vi "Raster_Scan_FSRS.vi"() -> ()   [LabVIEW 2014] (continued)
{"X"=544.0, "Y"=0.9978545183540273}, {"X"=545.0, "Y"=0.9978954802718253}, {"X"=546.0, "Y"=0.9978847126029841}, {"X"=547.0, "Y"=0.9986282274099947}, {"X"=548.0, "Y"=0.9985592746779094}, {"X"=549.0, "Y"=0.9984101644173519}, {"X"=550.0, "Y"=0.9981985424776665}, {"X"=551.0, "Y"=0.998426104497088}, {"X"=552.0, "Y"=0.9985691286987668}, {"X"=553.0, "Y"=0.9979689171383916}, {"X"=554.0, "Y"=0.9982460987713048}, {"X"=555.0, "Y"=0.998121473974186}, {"X"=556.0, "Y"=0.9977379675030132}, {"X"=557.0, "Y"=0.998243375619955}, {"X"=558.0, "Y"=0.998132359067814}, {"X"=559.0, "Y"=0.9983256230790136}, {"X"=560.0, "Y"=0.9980172261705131}, {"X"=561.0, "Y"=0.9984771190185349}, {"X"=562.0, "Y"=0.9979225481535584}, {"X"=563.0, "Y"=0.9981209325830508}, {"X"=564.0, "Y"=0.9981205014531911}, {"X"=565.0, "Y"=0.9985116348563284}, {"X"=566.0, "Y"=0.9985313300015474}, {"X"=567.0, "Y"=0.9985618507511264}, {"X"=568.0, "Y"=0.9980731056228417}, {"X"=569.0, "Y"=0.99777584834941}, {"X"=570.0, "Y"=0.9983204895779979}, {"X"=571.0, "Y"=0.9979093460943547}, {"X"=572.0, "Y"=0.9974202665539573}, {"X"=573.0, "Y"=0.9974138091852186}, {"X"=574.0, "Y"=0.99811669466617}, {"X"=575.0, "Y"=0.9981038738953151}, {"X"=576.0, "Y"=0.9977082372079878}, {"X"=577.0, "Y"=0.9980030461884963}, {"X"=578.0, "Y"=0.9980034114768427}, {"X"=579.0, "Y"=0.9982364510217848}, {"X"=580.0, "Y"=0.9979325576022529}, {"X"=581.0, "Y"=0.9977734094940269}, {"X"=582.0, "Y"=0.9981140314943433}, {"X"=583.0, "Y"=0.9979539107254143}, {"X"=584.0, "Y"=0.997655931871743}, {"X"=585.0, "Y"=0.9972543054374033}, {"X"=586.0, "Y"=0.9969317121833642}, {"X"=587.0, "Y"=0.9968443093625065}, {"X"=588.0, "Y"=0.9966413383535035}, {"X"=589.0, "Y"=0.9960249116592703}, {"X"=590.0, "Y"=0.9963089300738579}, {"X"=591.0, "Y"=0.9961840817664352}, {"X"=592.0, "Y"=0.9963553748195709}, {"X"=593.0, "Y"=0.9962705798119079}, {"X"=594.0, "Y"=0.99670571106408}, {"X"=595.0, "Y"=0.9964327341637447}, {"X"=596.0, "Y"=0.9965823060297267}, {"X"=597.0, "Y"=0.9968535449226337}, {"X"=598.0, "Y"=0.9965539588406062}, {"X"=599.0, "Y"=0.9961449417496469}, {"X"=600.0, "Y"=0.9965984047900572}, {"X"=601.0, "Y"=0.9962586900884038}, {"X"=602.0, "Y"=0.9962103374424071}, {"X"=603.0, "Y"=0.9954906975090069}, {"X"=604.0, "Y"=0.9957365549620107}, {"X"=605.0, "Y"=0.9963388156166715}, {"X"=606.0, "Y"=0.9965861993129}, {"X"=607.0, "Y"=0.9974232683784019}, {"X"=608.0, "Y"=0.9992020432658635}, {"X"=609.0, "Y"=1.00039405639493}, {"X"=610.0, "Y"=1.0013783401587335}, {"X"=611.0, "Y"=1.0033275791215845}, {"X"=612.0, "Y"=1.0047939581934993}, {"X"=613.0, "Y"=1.0072483446876968}, {"X"=614.0, "Y"=1.008871757151934}, {"X"=615.0, "Y"=1.0110282901417909}, {"X"=616.0, "Y"=1.013371337166815}, {"X"=617.0, "Y"=1.0151009747430668}, {"X"=618.0, "Y"=1.0176425122069255}, {"X"=619.0, "Y"=1.0197495431887913}, {"X"=620.0, "Y"=1.0224688407170561}, {"X"=621.0, "Y"=1.0247490900420204}, {"X"=622.0, "Y"=1.0276990459376787}, {"X"=623.0, "Y"=1.0296095041094517}, {"X"=624.0, "Y"=1.0333078315506532}, {"X"=625.0, "Y"=1.0362685626177792}, {"X"=626.0, "Y"=1.038924641533091}, {"X"=627.0, "Y"=1.041572265389145}, {"X"=628.0, "Y"=1.0435587138867348}, {"X"=629.0, "Y"=1.0464705907166}, {"X"=630.0, "Y"=1.0490032103492144}, {"X"=631.0, "Y"=1.050504978522211}, {"X"=632.0, "Y"=1.0528251069017325}, {"X"=633.0, "Y"=1.0534239144824968}, {"X"=634.0, "Y"=1.0549006626365562}, {"X"=635.0, "Y"=1.0550592680988555}, {"X"=636.0, "Y"=1.0549458189191194}, {"X"=637.0, "Y"=1.0549779342343906}, {"X"=638.0, "Y"=1.0539315349680067}, {"X"=639.0, "Y"=1.0542361563716711}, {"X"=640.0, "Y"=1.0534478719509481}, {"X"=641.0, "Y"=1.052399132550848}, {"X"=642.0, "Y"=1.0514082647686147}, {"X"=643.0, "Y"=1.0504137881143336}, {"X"=644.0, "Y"=1.0488047450457352}, {"X"=645.0, "Y"=1.0477270368509513}, {"X"=646.0, "Y"=1.045690156385211}, {"X"=647.0, "Y"=1.0432872265980713}, {"X"=648.0, "Y"=1.0410317960687832}, {"X"=649.0, "Y"=1.0379447532276453}, {"X"=650.0, "Y"=1.0348336539420064}, {"X"=651.0, "Y"=1.0315576847668324}, {"X"=652.0, "Y"=1.028862670120101}, {"X"=653.0, "Y"=1.0258567044055389}, {"X"=654.0, "Y"=1.0230131849598842}, {"X"=655.0, "Y"=1.0209637506857185}, {"X"=656.0, "Y"=1.0181556258277114}, {"X"=657.0, "Y"=1.0160814779436314}, {"X"=658.0, "Y"=1.0136796020817032}, {"X"=659.0, "Y"=1.0120789147322529}, {"X"=660.0, "Y"=1.0104539182883303}, {"X"=661.0, "Y"=1.008677968134813}, {"X"=662.0, "Y"=1.0068674140821063}, {"X"=663.0, "Y"=1.005416554572116}, {"X"=664.0, "Y"=1.004418287860281}, {"X"=665.0, "Y"=1.0026019255081793}, {"X"=666.0, "Y"=1.001755051681397}, {"X"=667.0, "Y"=1.0007427244836384}, {"X"=668.0, "Y"=1.000212255121392}, {"X"=669.0, "Y"=1.0001516680923108}, {"X"=670.0, "Y"=1.0002951868519772}, {"X"=671.0, "Y"=0.9997153062030121}, {"X"=672.0, "Y"=0.9996816416219783}, {"X"=673.0, "Y"=0.9998761682577347}, {"X"=674.0, "Y"=0.9992615693650128}, {"X"=675.0, "Y"=1.000324398030068}, {"X"=676.0, "Y"=0.9999570200209895}, {"X"=677.0, "Y"=1.0000117210295363}, {"X"=678.0, "Y"=1.0000634134316824}, {"X"=679.0, "Y"=1.0001331522973944}, {"X"=680.0, "Y"=1.0004081949275365}, {"X"=681.0, "Y"=0.9998829901655063}, {"X"=682.0, "Y"=1.000187544558325}, {"X"=683.0, "Y"=1.0003801314997531}, {"X"=684.0, "Y"=1.0003149177046684}, {"X"=685.0, "Y"=0.9998517079056821}, {"X"=686.0, "Y"=1.0004100893131052}, {"X"=687.0, "Y"=1.0000016158957639}, {"X"=688.0, "Y"=1.0006017898810222}, {"X"=689.0, "Y"=1.0005718409574569}, {"X"=690.0, "Y"=1.0007007698411632}, {"X"=691.0, "Y"=1.000506938601441}, {"X"=692.0, "Y"=1.0000772828380353}, {"X"=693.0, "Y"=1.0005686668319205}, {"X"=694.0, "Y"=1.0009164301763613}, {"X"=695.0, "Y"=1.0004825673685438}, {"X"=696.0, "Y"=1.000543465394958}, {"X"=697.0, "Y"=1.00084754089509}, {"X"=698.0, "Y"=1.0006573921442272}, {"X"=699.0, "Y"=1.0008281174083582}, {"X"=700.0, "Y"=1.001000500464312}, {"X"=701.0, "Y"=1.0005876920760894}, {"X"=702.0, "Y"=1.000993095286034}, {"X"=703.0, "Y"=1.00056708158604}, {"X"=704.0, "Y"=1.0006259107721924}, {"X"=705.0, "Y"=1.0007697612854025}, {"X"=706.0, "Y"=1.000978106387117}, {"X"=707.0, "Y"=1.0007664078085046}, {"X"=708.0, "Y"=1.0011454626210547}, {"X"=709.0, "Y"=1.0011091615448482}, {"X"=710.0, "Y"=1.001056081943534}, {"X"=711.0, "Y"=1.0012334014028355}, {"X"=712.0, "Y"=1.0011837250778726}, {"X"=713.0, "Y"=1.000916622339644}, {"X"=714.0, "Y"=1.0012569862720535}, {"X"=715.0, "Y"=1.0009918254170156}, {"X"=716.0, "Y"=1.0007201726153137}, {"X"=717.0, "Y"=1.0011288843771156}, {"X"=718.0, "Y"=1.0008681092115939}, {"X"=719.0, "Y"=1.0009798044664915}, {"X"=720.0, "Y"=1.001112027329558}, {"X"=721.0, "Y"=1.0010204159387182}, {"X"=722.0, "Y"=1.0006192087669428}, {"X"=723.0, "Y"=1.0012939973290147}, {"X"=724.0, "Y"=1.0007005394153075}, {"X"=725.0, "Y"=1.0009357538518868}, {"X"=726.0, "Y"=1.0014740988896245}, {"X"=727.0, "Y"=1.0010121967650842}, {"X"=728.0, "Y"=1.0016954160298988}, {"X"=729.0, "Y"=1.0011144874969538}, {"X"=730.0, "Y"=1.000975865976058}, {"X"=731.0, "Y"=1.0011789828226225}, {"X"=732.0, "Y"=1.0011893085482935}, {"X"=733.0, "Y"=1.0011614230048504}, {"X"=734.0, "Y"=1.0011976845828305}, {"X"=735.0, "Y"=1.0011581305715418}, {"X"=736.0, "Y"=1.0010556075044197}, {"X"=737.0, "Y"=1.000937577300871}, {"X"=738.0, "Y"=1.0009325997585012}, {"X"=739.0, "Y"=1.0007734996223567}, {"X"=740.0, "Y"=1.0008682847275774}, {"X"=741.0, "Y"=1.0009267272013356}, {"X"=742.0, "Y"=1.0009202446313439}, {"X"=743.0, "Y"=1.0011286199467828}, {"X"=744.0, "Y"=1.0009420307972523}, {"X"=745.0, "Y"=1.0011039647090711}, {"X"=746.0, "Y"=1.0009233724169802}, {"X"=747.0, "Y"=1.0007503724260123}, {"X"=748.0, "Y"=1.0008308485115536}, {"X"=749.0, "Y"=1.0009287533631965}, {"X"=750.0, "Y"=1.0007719252489964}, {"X"=751.0, "Y"=1.0008692070915899}, {"X"=752.0, "Y"=1.0008582123092458}, {"X"=753.0, "Y"=1.0005798712787062}, {"X"=754.0, "Y"=1.0009749912624057}, {"X"=755.0, "Y"=1.0009132421180837}, {"X"=756.0, "Y"=1.0006067695791088}, {"X"=757.0, "Y"=1.0006890331168343}, {"X"=758.0, "Y"=1.0008962054677861}, {"X"=759.0, "Y"=1.0005844554606693}, {"X"=760.0, "Y"=1.0008238897141335}, {"X"=761.0, "Y"=1.0008713716200581}, {"X"=762.0, "Y"=1.000462698368419}, {"X"=763.0, "Y"=1.00038551560003}, {"X"=764.0, "Y"=1.0005740364073854}, {"X"=765.0, "Y"=1.0010253429662304}, {"X"=766.0, "Y"=1.0003632657418395}, {"X"=767.0, "Y"=1.000567308693705}, {"X"=768.0, "Y"=1.000286790348577}, {"X"=769.0, "Y"=1.0004665761914815}, {"X"=770.0, "Y"=1.000168483840905}, {"X"=771.0, "Y"=1.000152637463018}, {"X"=772.0, "Y"=1.000214242192368}, {"X"=773.0, "Y"=1.0003869867588742}, {"X"=774.0, "Y"=1.0005376955714191}, {"X"=775.0, "Y"=1.0004800558745468}, {"X"=776.0, "Y"=1.0005707911790136}, {"X"=777.0, "Y"=0.9997487173368662}, {"X"=778.0, "Y"=1.0004505353589024}, {"X"=779.0, "Y"=1.0006358048732418}, {"X"=780.0, "Y"=1.0006913500666466}, {"X"=781.0, "Y"=1.0000594857246996}, {"X"=782.0, "Y"=1.000202033665066}, {"X"=783.0, "Y"=1.0005896258602271}, {"X"=784.0, "Y"=0.9998116953891122}, {"X"=785.0, "Y"=1.0000030368836728}, {"X"=786.0, "Y"=0.9999692468282858}, {"X"=787.0, "Y"=0.9996749236190133}, {"X"=788.0, "Y"=0.9999528813725637}, {"X"=789.0, "Y"=0.9996934968232128}, {"X"=790.0, "Y"=1.0001246386179192}, {"X"=791.0, "Y"=1.000121231707337}, {"X"=792.0, "Y"=1.0003574387962126}, {"X"=793.0, "Y"=0.9998897647562817}, {"X"=794.0, "Y"=0.999991814875864}, {"X"=795.0, "Y"=0.9999717796372998}, {"X"=796.0, "Y"=0.9999164248339153}, {"X"=797.0, "Y"=1.0000472803501612}, {"X"=798.0, "Y"=1.0003096307675872}, {"X"=799.0, "Y"=0.9995521439215307}, {"X"=800.0, "Y"=0.9998268441921865}, {"X"=801.0, "Y"=0.9997823002205563}, {"X"=802.0, "Y"=0.9997914401002861}, {"X"=803.0, "Y"=0.999436665219622}, {"X"=804.0, "Y"=0.9996389638963711}, {"X"=805.0, "Y"=0.999683035386018}, {"X"=806.0, "Y"=0.9999043749665063}, {"X"=807.0, "Y"=0.999872375868445}, {"X"=808.0, "Y"=0.9995564412851898}, {"X"=809.0, "Y"=0.9997146784363528}, {"X"=810.0, "Y"=0.9992468990944221}, {"X"=811.0, "Y"=0.9999100681507468}, {"X"=812.0, "Y"=0.9996803844051546}, {"X"=813.0, "Y"=0.999812736922049}, {"X"=814.0, "Y"=0.9999079641000937}, {"X"=815.0, "Y"=0.9995712757348625}, {"X"=816.0, "Y"=0.9999753952150852}, {"X"=817.0, "Y"=0.9996161230527898}, {"X"=818.0, "Y"=0.9999692827506793}, {"X"=819.0, "Y"=0.9997854374958309}, {"X"=820.0, "Y"=0.9997379623488489}, {"X"=821.0, "Y"=0.9997951408693897}, {"X"=822.0, "Y"=0.9996005558855302}, {"X"=823.0, "Y"=0.9996013042279536}, {"X"=824.0, "Y"=0.9994527699487141}, {"X"=825.0, "Y"=0.9994611971332913}, {"X"=826.0, "Y"=0.9995943046267404}, {"X"=827.0, "Y"=0.9993996315141247}, {"X"=828.0, "Y"=0.999466764473007}, {"X"=829.0, "Y"=0.9997275186993784}, {"X"=830.0, "Y"=0.9994655220422562}, {"X"=831.0, "Y"=0.9999217304306618}, {"X"=832.0, "Y"=0.9995485361962716}, {"X"=833.0, "Y"=0.9998723066127978}, {"X"=834.0, "Y"=0.9995042794915885}, {"X"=835.0, "Y"=0.9995245056820103}, {"X"=836.0, "Y"=0.9991550561955388}, {"X"=837.0, "Y"=0.9996330482905573}, {"X"=838.0, "Y"=0.9999634602317182}, {"X"=839.0, "Y"=0.999554498145934}, {"X"=840.0, "Y"=0.9993969166206773}, {"X"=841.0, "Y"=0.9994570922088231}, {"X"=842.0, "Y"=0.9994160747857141}, {"X"=843.0, "Y"=0.9995563480657043}, {"X"=844.0, "Y"=0.9999575192332566}, {"X"=845.0, "Y"=0.9994287267946973}, {"X"=846.0, "Y"=0.9997828708624986}, {"X"=847.0, "Y"=0.9997294658304303}, {"X"=848.0, "Y"=0.9997987491676308}, {"X"=849.0, "Y"=0.9998366805189256}, {"X"=850.0, "Y"=0.9998421980321909}, {"X"=851.0, "Y"=0.9997708290381001}, {"X"=852.0, "Y"=0.9997571893188337}, {"X"=853.0, "Y"=0.9999425601459052}, {"X"=854.0, "Y"=0.999591626867619}, {"X"=855.0, "Y"=0.9997575945123861}, {"X"=856.0, "Y"=0.9998259214523023}, {"X"=857.0, "Y"=0.9998524142922023}, {"X"=858.0, "Y"=0.9998214349671982}, {"X"=859.0, "Y"=0.9996982431382163}, {"X"=860.0, "Y"=1.000006724215444}, {"X"=861.0, "Y"=0.9997226946982664}, {"X"=862.0, "Y"=1.0001222798385383}, {"X"=863.0, "Y"=0.9997723680899672}, {"X"=864.0, "Y"=1.0004691521323734}, {"X"=865.0, "Y"=0.9995317329722564}, {"X"=866.0, "Y"=0.9999706638370606}, {"X"=867.0, "Y"=0.9999485081385426}, {"X"=868.0, "Y"=1.0002513015681866}, {"X"=869.0, "Y"=1.0001094834288995}, {"X"=870.0, "Y"=1.0000796165289747}, {"X"=871.0, "Y"=1.0001052236277999}, {"X"=872.0, "Y"=1.0004937362292834}, {"X"=873.0, "Y"=1.000013590642817}, {"X"=874.0, "Y"=1.0003573287643348}, {"X"=875.0, "Y"=1.0004525481711148}, {"X"=876.0, "Y"=0.9999755900094128}, {"X"=877.0, "Y"=1.0003964124631561}, {"X"=878.0, "Y"=1.0005363708541122}, {"X"=879.0, "Y"=1.0004557806466459}, {"X"=880.0, "Y"=1.000733510349076}, {"X"=881.0, "Y"=1.0002652087127946}, {"X"=882.0, "Y"=1.0003971179645745}, {"X"=883.0, "Y"=1.0006048161778602}, {"X"=884.0, "Y"=1.0005937878882152}, {"X"=885.0, "Y"=1.000476561139529}, {"X"=886.0, "Y"=1.0004827953448545}, {"X"=887.0, "Y"=1.000421392196533}, {"X"=888.0, "Y"=1.0003776494746428}, {"X"=889.0, "Y"=1.0002335494105024}, {"X"=890.0, "Y"=1.0005818770177213}, {"X"=891.0, "Y"=1.000556169743754}, {"X"=892.0, "Y"=1.0005142471348096}, {"X"=893.0, "Y"=1.0006009804720526}, {"X"=894.0, "Y"=1.000462567319067}, {"X"=895.0, "Y"=1.0004232511191642}, {"X"=896.0, "Y"=1.0002985391510821}, {"X"=897.0, "Y"=1.000563080763287}, {"X"=898.0, "Y"=1.0003985868488332}, {"X"=899.0, "Y"=1.0005921693519613}, {"X"=900.0, "Y"=1.0005517113896354}, {"X"=901.0, "Y"=1.0004511874507864}, {"X"=902.0, "Y"=1.0003164509105338}, {"X"=903.0, "Y"=1.0006514699992903}, {"X"=904.0, "Y"=1.0004630517353699}, {"X"=905.0, "Y"=1.0003696899849848}, {"X"=906.0, "Y"=1.0000750343598261}, {"X"=907.0, "Y"=1.0001652803283667}, {"X"=908.0, "Y"=1.0005821961595347}, {"X"=909.0, "Y"=1.0000753056610996}, {"X"=910.0, "Y"=1.0008381429666606}, {"X"=911.0, "Y"=1.0002009630275162}, {"X"=912.0, "Y"=1.0000090046202812}, {"X"=913.0, "Y"=1.000357217161673}, {"X"=914.0, "Y"=1.0005551947210591}, {"X"=915.0, "Y"=1.0006019344688362}, {"X"=916.0, "Y"=1.0003157102839864}, {"X"=917.0, "Y"=1.0006539638821532}, {"X"=918.0, "Y"=1.0004523550286122}, {"X"=919.0, "Y"=1.0004362081948674}, {"X"=920.0, "Y"=1.0004658381122902}, {"X"=921.0, "Y"=1.0005032431132526}, {"X"=922.0, "Y"=1.0006496135004674}, {"X"=923.0, "Y"=1.000421409515476}, {"X"=924.0, "Y"=1.00029741571484}, {"X"=925.0, "Y"=1.0003752604308016}, {"X"=926.0, "Y"=1.0000674401177483}, {"X"=927.0, "Y"=1.000752504898771}, {"X"=928.0, "Y"=1.0004265589119117}, {"X"=929.0, "Y"=1.000277485793791}, {"X"=930.0, "Y"=1.000143732812286}, {"X"=931.0, "Y"=1.000586072623539}, {"X"=932.0, "Y"=1.0003218460655414}, {"X"=933.0, "Y"=1.000253779745408}, {"X"=934.0, "Y"=0.9999684895073191}, {"X"=935.0, "Y"=1.0000553542910315}, {"X"=936.0, "Y"=1.0004387435193063}, {"X"=937.0, "Y"=1.0005796043709154}, {"X"=938.0, "Y"=1.0002239035981928}, {"X"=939.0, "Y"=1.0005100497007755}, {"X"=940.0, "Y"=1.000276926115426}, {"X"=941.0, "Y"=1.0005393916224292}, {"X"=942.0, "Y"=1.0003102290640964}, {"X"=943.0, "Y"=1.0004510828201474}, {"X"=944.0, "Y"=1.0004024270555596}, {"X"=945.0, "Y"=1.0003071722234138}, {"X"=946.0, "Y"=1.0003479438286045}, {"X"=947.0, "Y"=1.0006054265939661}, {"X"=948.0, "Y"=1.0004341205130898}, {"X"=949.0, "Y"=1.0005543120812839}, {"X"=950.0, "Y"=1.0004009168011205}, {"X"=951.0, "Y"=1.0006692411711766}, {"X"=952.0, "Y"=1.0005684966442148}, {"X"=953.0, "Y"=1.0002059600051625}, {"X"=954.0, "Y"=1.0004913192089357}, {"X"=955.0, "Y"=1.0003185704962576}, {"X"=956.0, "Y"=1.0003571139773684}, {"X"=957.0, "Y"=1.0004792329148344}, {"X"=958.0, "Y"=1.0007107646312456}, {"X"=959.0, "Y"=1.0003472703541094}, {"X"=960.0, "Y"=1.00055060436529}, {"X"=961.0, "Y"=1.0002969671654476}, {"X"=962.0, "Y"=1.0002867873822994}, {"X"=963.0, "Y"=1.0003786420047431}, {"X"=964.0, "Y"=1.0003682377805028}, {"X"=965.0, "Y"=1.0005896761650959}, {"X"=966.0, "Y"=1.0003457782727248}, {"X"=967.0, "Y"=1.0006909634949526}, {"X"=968.0, "Y"=1.0001113405044946}, {"X"=969.0, "Y"=1.0003299278640605}, {"X"=970.0, "Y"=1.0006022370584085}, {"X"=971.0, "Y"=1.0002903312662772}, {"X"=972.0, "Y"=1.0005061770542671}, {"X"=973.0, "Y"=1.0004220088897762}, {"X"=974.0, "Y"=1.00062971722216}, {"X"=975.0, "Y"=1.0003765492341081}, {"X"=976.0, "Y"=1.0004592871043285}, {"X"=977.0, "Y"=1.000514847516494}, {"X"=978.0, "Y"=1.0003467113971076}, {"X"=979.0, "Y"=1.0002069450901978}, {"X"=980.0, "Y"=1.0005040498159148}, {"X"=981.0, "Y"=1.000138336954979}, {"X"=982.0, "Y"=1.000390235537673}, {"X"=983.0, "Y"=1.000504818092738}, {"X"=984.0, "Y"=1.0002436968618853}, {"X"=985.0, "Y"=1.0004223209898575}, {"X"=986.0, "Y"=1.0002155513016582}, {"X"=987.0, "Y"=1.0001190993872675}, {"X"=988.0, "Y"=1.000394310225494}, {"X"=989.0, "Y"=1.0004553646966243}, {"X"=990.0, "Y"=1.0001042595318252}, {"X"=991.0, "Y"=1.000235823625573}, {"X"=992.0, "Y"=1.0002616383711564}, {"X"=993.0, "Y"=1.0003022919280078}, {"X"=994.0, "Y"=1.000557447133573}, {"X"=995.0, "Y"=1.0002431232712843}, {"X"=996.0, "Y"=1.000407779249664}, {"X"=997.0, "Y"=1.0001910030091277}, {"X"=998.0, "Y"=1.0000811448918354}, {"X"=999.0, "Y"=1.000409690537901}, {"X"=1000.0, "Y"=1.0003398218940822}, {"X"=1001.0, "Y"=1.000204245610935}, {"X"=1002.0, "Y"=1.00018533413993}, {"X"=1003.0, "Y"=1.000302314225904}, {"X"=1004.0, "Y"=1.0002923742421739}, {"X"=1005.0, "Y"=1.000309364574194}, {"X"=1006.0, "Y"=1.0000426923874066}, {"X"=1007.0, "Y"=1.0004618206725626}, {"X"=1008.0, "Y"=1.0003141108219815}, {"X"=1009.0, "Y"=1.0005023576969727}, {"X"=1010.0, "Y"=1.0003544772082134}, {"X"=1011.0, "Y"=1.0004524090568325}, {"X"=1012.0, "Y"=1.0001465182625013}, {"X"=1013.0, "Y"=1.0002729209887085}, {"X"=1014.0, "Y"=1.0003807048184004}, {"X"=1015.0, "Y"=1.0000934145436753}, {"X"=1016.0, "Y"=1.000523744822201}, {"X"=1017.0, "Y"=1.0003810050685418}, {"X"=1018.0, "Y"=1.0001897441615633}, {"X"=1019.0, "Y"=1.0000433790093919}, {"X"=1020.0, "Y"=1.0002344668735443}, {"X"=1021.0, "Y"=1.0000743430369654}, {"X"=1022.0, "Y"=1.0005123321725913}, {"X"=1023.0, "Y"=0.9999867984833275}, {"X"=1024.0, "Y"=1.00028886416398}, {"X"=1025.0, "Y"=0.9999976564025252}, {"X"=1026.0, "Y"=1.000147489191159}, {"X"=1027.0, "Y"=1.0001021283303542}, {"X"=1028.0, "Y"=1.0004207742794315}, {"X"=1029.0, "Y"=1.0003511315237172}, {"X"=1030.0, "Y"=1.0002740488978419}, {"X"=1031.0, "Y"=1.0005715604928058}, {"X"=1032.0, "Y"=1.0000849731377497}, {"X"=1033.0, "Y"=1.000664325326948}, {"X"=1034.0, "Y"=1.0002715158858457}, {"X"=1035.0, "Y"=1.0004068426842052}, {"X"=1036.0, "Y"=1.0003341226908409}, {"X"=1037.0, "Y"=1.0003845014598438}, {"X"=1038.0, "Y"=1.000382059982626}, {"X"=1039.0, "Y"=1.0002566925098917}, {"X"=1040.0, "Y"=1.0004394237268197}, {"X"=1041.0, "Y"=1.0003796791309603}, {"X"=1042.0, "Y"=1.0005573908410998}, {"X"=1043.0, "Y"=1.0003274420534478}, {"X"=1044.0, "Y"=1.000649864733999}, {"X"=1045.0, "Y"=1.0001894757842382}, {"X"=1046.0, "Y"=1.0003630377518922}, {"X"=1047.0, "Y"=1.0007311125223617}, {"X"=1048.0, "Y"=1.0003937967302898}, {"X"=1049.0, "Y"=1.0004660000627263}, {"X"=1050.0, "Y"=1.000370743171769}, {"X"=1051.0, "Y"=1.0003895018697897}, {"X"=1052.0, "Y"=1.0003660457840664}, {"X"=1053.0, "Y"=1.0006618337709967}, {"X"=1054.0, "Y"=1.0004746367542625}, {"X"=1055.0, "Y"=1.0006470220462966}, {"X"=1056.0, "Y"=1.000336358127014}, {"X"=1057.0, "Y"=1.0004776161543254}, {"X"=1058.0, "Y"=1.0005350625396425}, {"X"=1059.0, "Y"=1.0007114086431932}, {"X"=1060.0, "Y"=1.0005461150814388}, {"X"=1061.0, "Y"=1.0001568330212558}, {"X"=1062.0, "Y"=1.0006049675270903}, {"X"=1063.0, "Y"=1.0008072532845746}, {"X"=1064.0, "Y"=1.0007899340972959}, {"X"=1065.0, "Y"=1.0003705264800233}, {"X"=1066.0, "Y"=1.000663501831443}, {"X"=1067.0, "Y"=1.0003968148498383}, {"X"=1068.0, "Y"=1.0004410295865593}, {"X"=1069.0, "Y"=1.000990825072581}, {"X"=1070.0, "Y"=1.0007069226291818}, {"X"=1071.0, "Y"=1.0009074944245333}, {"X"=1072.0, "Y"=1.000986596814561}, {"X"=1073.0, "Y"=1.0006469461319005}, {"X"=1074.0, "Y"=1.0006961161864978}, {"X"=1075.0, "Y"=1.0009206991231543}, {"X"=1076.0, "Y"=1.0004970130469557}, {"X"=1077.0, "Y"=1.0008897415638358}, {"X"=1078.0, "Y"=1.0004689157169488}, {"X"=1079.0, "Y"=1.0008271789537952}, {"X"=1080.0, "Y"=1.0005958642457493}, {"X"=1081.0, "Y"=1.0006627201543532}, {"X"=1082.0, "Y"=1.000911669123488}, {"X"=1083.0, "Y"=1.0007669752129835}, {"X"=1084.0, "Y"=1.0007869594284737}, {"X"=1085.0, "Y"=1.0008017239957097}, {"X"=1086.0, "Y"=1.0006641645030927}, {"X"=1087.0, "Y"=1.0004027285217332}, {"X"=1088.0, "Y"=1.0005489411934159}, {"X"=1089.0, "Y"=1.0007225000918056}, {"X"=1090.0, "Y"=1.0009034474609535}, {"X"=1091.0, "Y"=1.000700412495902}, {"X"=1092.0, "Y"=1.000559530919639}, {"X"=1093.0, "Y"=1.000504483593376}, {"X"=1094.0, "Y"=1.0006442407338632}, {"X"=1095.0, "Y"=1.0007664841012642}, {"X"=1096.0, "Y"=1.000595386528809}, {"X"=1097.0, "Y"=1.0006037218552855}, {"X"=1098.0, "Y"=1.0006076992023385}, {"X"=1099.0, "Y"=1.0008559458938961}, {"X"=1100.0, "Y"=1.0003974508855653}, {"X"=1101.0, "Y"=1.000520661832493}, {"X"=1102.0, "Y"=1.0007578111149742}, {"X"=1103.0, "Y"=1.0008950719357999}, {"X"=1104.0, "Y"=1.0005845587993554}, {"X"=1105.0, "Y"=1.0004975573787183}, {"X"=1106.0, "Y"=1.0005630280187985}, {"X"=1107.0, "Y"=1.0004865609128089}, {"X"=1108.0, "Y"=1.0005512637747156}, {"X"=1109.0, "Y"=1.0002904477140733}, {"X"=1110.0, "Y"=1.0007674753310123}, {"X"=1111.0, "Y"=1.00048425912666}, {"X"=1112.0, "Y"=1.000537310412031}, {"X"=1113.0, "Y"=1.0003184257671687}, {"X"=1114.0, "Y"=1.000551378960108}, {"X"=1115.0, "Y"=1.0004538385686341}, {"X"=1116.0, "Y"=1.0004718054037691}, {"X"=1117.0, "Y"=1.0005247856359447}, {"X"=1118.0, "Y"=1.000659286030276}, {"X"=1119.0, "Y"=1.0005952741982334}, {"X"=1120.0, "Y"=1.0003527948470332}, {"X"=1121.0, "Y"=1.0003785102284437}, {"X"=1122.0, "Y"=1.0003192400893162}, {"X"=1123.0, "Y"=1.0003699743364536}, {"X"=1124.0, "Y"=1.0004382463116217}, {"X"=1125.0, "Y"=1.0006464169345477}, {"X"=1126.0, "Y"=1.000249392202887}, {"X"=1127.0, "Y"=1.0003913257192574}, {"X"=1128.0, "Y"=1.0002131029939758}, {"X"=1129.0, "Y"=1.000510325890708}, {"X"=1130.0, "Y"=1.0003934905817833}, {"X"=1131.0, "Y"=1.0004037059793067}, {"X"=1132.0, "Y"=1.0006618492578454}, {"X"=1133.0, "Y"=1.0003001585452074}, {"X"=1134.0, "Y"=1.000318694948343}, {"X"=1135.0, "Y"=1.000487815893616}, {"X"=1136.0, "Y"=1.0003780216915208}, {"X"=1137.0, "Y"=1.000413317598835}, {"X"=1138.0, "Y"=1.0002135307505462}, {"X"=1139.0, "Y"=1.0003336207033005}, {"X"=1140.0, "Y"=1.000519988073343}, {"X"=1141.0, "Y"=1.000548679843787}, {"X"=1142.0, "Y"=1.000496056734601}, {"X"=1143.0, "Y"=1.0004444345976555}, {"X"=1144.0, "Y"=1.0001817232823744}, {"X"=1145.0, "Y"=1.000174005105797}, {"X"=1146.0, "Y"=1.000292447162328}, {"X"=1147.0, "Y"=1.0003638645546393}, {"X"=1148.0, "Y"=1.0002355752060164}, {"X"=1149.0, "Y"=1.00033455515827}, {"X"=1150.0, "Y"=1.0003245306564827}, {"X"=1151.0, "Y"=1.0002618152857234}, {"X"=1152.0, "Y"=1.0002737777366781}, {"X"=1153.0, "Y"=1.0002170643978059}, {"X"=1154.0, "Y"=1.000413604154719}, {"X"=1155.0, "Y"=1.0003099390465664}, {"X"=1156.0, "Y"=1.0005132182782912}, {"X"=1157.0, "Y"=1.000114107216987}, {"X"=1158.0, "Y"=1.0004770062354829}, {"X"=1159.0, "Y"=1.0004171034572575}, {"X"=1160.0, "Y"=1.0004569184938314}, {"X"=1161.0, "Y"=1.0004500384099237}, {"X"=1162.0, "Y"=1.0003170786145168}, {"X"=1163.0, "Y"=1.0002788252400026}, {"X"=1164.0, "Y"=1.0001948307072348}, {"X"=1165.0, "Y"=1.000410823030397}, {"X"=1166.0, "Y"=1.0004580665102198}, {"X"=1167.0, "Y"=1.0006692310587075}, {"X"=1168.0, "Y"=1.0003228737956749}, {"X"=1169.0, "Y"=1.0004916680510918}, {"X"=1170.0, "Y"=1.0003407364670853}, {"X"=1171.0, "Y"=1.0004045567333217}, {"X"=1172.0, "Y"=1.0003803654908978}, {"X"=1173.0, "Y"=1.0005615371076164}, {"X"=1174.0, "Y"=1.0004756109300434}, {"X"=1175.0, "Y"=1.0002314936984527}, {"X"=1176.0, "Y"=1.0004712973824592}, {"X"=1177.0, "Y"=1.0004057411969836}, {"X"=1178.0, "Y"=1.000628559692479}, {"X"=1179.0, "Y"=1.0003217635313526}, {"X"=1180.0, "Y"=1.0005789076417058}, {"X"=1181.0, "Y"=1.0004029462741326}, {"X"=1182.0, "Y"=1.0004755736162572}, {"X"=1183.0, "Y"=1.000328213200497}, {"X"=1184.0, "Y"=1.0003231498600846}, {"X"=1185.0, "Y"=1.000319103874417}, {"X"=1186.0, "Y"=1.0003228774765789}, {"X"=1187.0, "Y"=1.0003140546407656}, {"X"=1188.0, "Y"=1.0002848343336417}, {"X"=1189.0, "Y"=1.000508203882091}, {"X"=1190.0, "Y"=1.0002593068654488}, {"X"=1191.0, "Y"=1.000528935806764}, {"X"=1192.0, "Y"=1.0002378049460148}, {"X"=1193.0, "Y"=1.0005706812105148}, {"X"=1194.0, "Y"=1.0005374034632506}, {"X"=1195.0, "Y"=1.0001988163757602}, {"X"=1196.0, "Y"=1.0006119463054979}, {"X"=1197.0, "Y"=1.0004849225241381}, {"X"=1198.0, "Y"=1.0001640223128738}, {"X"=1199.0, "Y"=1.000498524564885}, {"X"=1200.0, "Y"=1.0004647778536588}, {"X"=1201.0, "Y"=1.000694727887658}, {"X"=1202.0, "Y"=1.0005207959941573}, {"X"=1203.0, "Y"=1.0004819931045297}, {"X"=1204.0, "Y"=1.000408028714742}, {"X"=1205.0, "Y"=1.000452772334067}, {"X"=1206.0, "Y"=1.0004315291178194}, {"X"=1207.0, "Y"=1.000614562289016}, {"X"=1208.0, "Y"=1.0004267608269495}, {"X"=1209.0, "Y"=1.0005413247966406}, {"X"=1210.0, "Y"=1.0003336212758853}, {"X"=1211.0, "Y"=1.0005233093467742}, {"X"=1212.0, "Y"=1.0001841951286268}, {"X"=1213.0, "Y"=1.000496276064622}, {"X"=1214.0, "Y"=1.0004435113554953}, {"X"=1215.0, "Y"=1.000312762889553}, {"X"=1216.0, "Y"=1.0003880506852765}, {"X"=1217.0, "Y"=1.0004430152993407}, {"X"=1218.0, "Y"=1.0005048604950806}, {"X"=1219.0, "Y"=1.0005918812246315}, {"X"=1220.0, "Y"=1.0005451398371954}, {"X"=1221.0, "Y"=1.0003538628812572}, {"X"=1222.0, "Y"=1.0002957581328165}, {"X"=1223.0, "Y"=1.0003455069942162}, {"X"=1224.0, "Y"=1.000559760984321}, {"X"=1225.0, "Y"=1.0006259813372131}, {"X"=1226.0, "Y"=1.0005780148556396}, {"X"=1227.0, "Y"=1.000428860631512}, {"X"=1228.0, "Y"=1.0003284274537925}, {"X"=1229.0, "Y"=1.0003759087401576}, {"X"=1230.0, "Y"=1.0004160325486642}, {"X"=1231.0, "Y"=1.000516966469858}, {"X"=1232.0, "Y"=1.0003531105538244}, {"X"=1233.0, "Y"=1.0003040660663642}, {"X"=1234.0, "Y"=1.0002145369130029}, {"X"=1235.0, "Y"=1.0006000845056313}, {"X"=1236.0, "Y"=1.0001780143915535}, {"X"=1237.0, "Y"=1.000413099776387}, {"X"=1238.0, "Y"=1.000340814364807}, {"X"=1239.0, "Y"=1.0003847961728747}, {"X"=1240.0, "Y"=1.0003377689644548}, {"X"=1241.0, "Y"=1.000235110479406}, {"X"=1242.0, "Y"=1.0003788090882357}, {"X"=1243.0, "Y"=1.0002683715599725}, {"X"=1244.0, "Y"=1.0005668734989672}, {"X"=1245.0, "Y"=1.0003983214098358}, {"X"=1246.0, "Y"=1.0004392908564488}, {"X"=1247.0, "Y"=1.0003490703578124}, {"X"=1248.0, "Y"=1.000515061423131}, {"X"=1249.0, "Y"=1.000536082836616}, {"X"=1250.0, "Y"=1.0006033938395056}, {"X"=1251.0, "Y"=1.000302436999363}, {"X"=1252.0, "Y"=1.0003435968686736}, {"X"=1253.0, "Y"=1.0003651518565015}, {"X"=1254.0, "Y"=1.0003753816897634}, {"X"=1255.0, "Y"=1.0004164707875218}, {"X"=1256.0, "Y"=1.0003124339083862}, {"X"=1257.0, "Y"=1.0006060617434724}, {"X"=1258.0, "Y"=1.0002433038607497}, {"X"=1259.0, "Y"=1.0005616162726159}, {"X"=1260.0, "Y"=1.0001358996051335}, {"X"=1261.0, "Y"=1.0004996326881244}, {"X"=1262.0, "Y"=1.000400823722666}, {"X"=1263.0, "Y"=1.0004651302016123}, {"X"=1264.0, "Y"=1.0004929661841928}, {"X"=1265.0, "Y"=1.000289786751315}, {"X"=1266.0, "Y"=1.0007068294577364}, {"X"=1267.0, "Y"=1.000512591719354}, {"X"=1268.0, "Y"=1.0005384306699427}, {"X"=1269.0, "Y"=1.000517410690437}, {"X"=1270.0, "Y"=1.0004457834676075}, {"X"=1271.0, "Y"=1.0003882566144624}, {"X"=1272.0, "Y"=1.000350183325496}, {"X"=1273.0, "Y"=1.0006835941128598}, {"X"=1274.0, "Y"=1.000354784112539}, {"X"=1275.0, "Y"=1.0005457804752032}, {"X"=1276.0, "Y"=1.0004234559458807}, {"X"=1277.0, "Y"=1.000496135909765}, {"X"=1278.0, "Y"=1.0002670384407588}, {"X"=1279.0, "Y"=1.0006040819275774}, {"X"=1280.0, "Y"=1.0002955765486259}, {"X"=1281.0, "Y"=1.000449882926412}, {"X"=1282.0, "Y"=1.000341046704705}, {"X"=1283.0, "Y"=1.0002621866108508}, {"X"=1284.0, "Y"=1.0002533451242017}, {"X"=1285.0, "Y"=1.0005020999666248}, {"X"=1286.0, "Y"=1.0004683221869657}, {"X"=1287.0, "Y"=1.0001189169044085}, {"X"=1288.0, "Y"=1.000394207742366}, {"X"=1289.0, "Y"=1.0004025113742172}, {"X"=1290.0, "Y"=1.0003591461387191}, {"X"=1291.0, "Y"=1.0002694424348582}, {"X"=1292.0, "Y"=1.000211944479205}, {"X"=1293.0, "Y"=1.0004554645660035}, {"X"=1294.0, "Y"=1.0004598057481355}, {"X"=1295.0, "Y"=1.0003228478676573}, {"X"=1296.0, "Y"=1.000281777127627}, {"X"=1297.0, "Y"=1.0003787502855446}, {"X"=1298.0, "Y"=1.0002643271177996}, {"X"=1299.0, "Y"=1.0003769449091497}, {"X"=1300.0, "Y"=1.0002871629718717}, {"X"=1301.0, "Y"=1.0002870790211043}, {"X"=1302.0, "Y"=1.0004704503723805}, {"X"=1303.0, "Y"=1.000476260657746}, {"X"=1304.0, "Y"=1.0004436163087576}, {"X"=1305.0, "Y"=1.0003863290955655}, {"X"=1306.0, "Y"=1.0005161647862937}, {"X"=1307.0, "Y"=1.0002249935131708}, {"X"=1308.0, "Y"=1.0005432839193034}, {"X"=1309.0, "Y"=1.0002816770022227}, {"X"=1310.0, "Y"=1.0004166737347884}, {"X"=1311.0, "Y"=1.000377784099795}, {"X"=1312.0, "Y"=1.000352088235326}, {"X"=1313.0, "Y"=1.0002378301300934}, {"X"=1314.0, "Y"=1.0004637548937716}, {"X"=1315.0, "Y"=1.0005468342453412}, {"X"=1316.0, "Y"=1.0002633492264565}, {"X"=1317.0, "Y"=1.000564439873648}, {"X"=1318.0, "Y"=1.0001624654733714}, {"X"=1319.0, "Y"=1.000511231090866}, {"X"=1320.0, "Y"=1.0003544601208683}, {"X"=1321.0, "Y"=1.0004053585602486}, {"X"=1322.0, "Y"=1.0004871315290047}, {"X"=1323.0, "Y"=1.0004300315929238}, {"X"=1324.0, "Y"=1.0003519445352231}, {"X"=1325.0, "Y"=1.0001932579752508}, {"X"=1326.0, "Y"=1.0004275604256458}, {"X"=1327.0, "Y"=1.0004909106276227}, {"X"=1328.0, "Y"=1.0003410593503033}, {"X"=1329.0, "Y"=1.0004439501902358}, {"X"=1330.0, "Y"=1.0005001161868323}, {"X"=1331.0, "Y"=1.0003332716770454}, {"X"=1332.0, "Y"=1.0005933376920328}, {"X"=1333.0, "Y"=1.0002798326870992}, {"X"=1334.0, "Y"=1.0004522633871564}, {"X"=1335.0, "Y"=1.0003822332936998}, {"X"=1336.0, "Y"=1.000511062012222}, {"X"=1337.0, "Y"=1.000358823903489}, {"X"=1338.0, "Y"=1.0006280323541772}, {"X"=1339.0, "Y"=1.00037812862855}]
  in  "# Images":u16=200 min=2 max=10000 step=2
  out "error out":errorcluster
  out "Camera Handle":u32=16842752
  out "Temperature":dbl=-75.5
  in  "error in":errorcluster
  # "Delay Stage Control"
  # "Calibration parameters"
  # "File Destination"
  # "Raster Scan Parameters"
  # "Microscope Stage Control"
  # "Fitting Parameters"
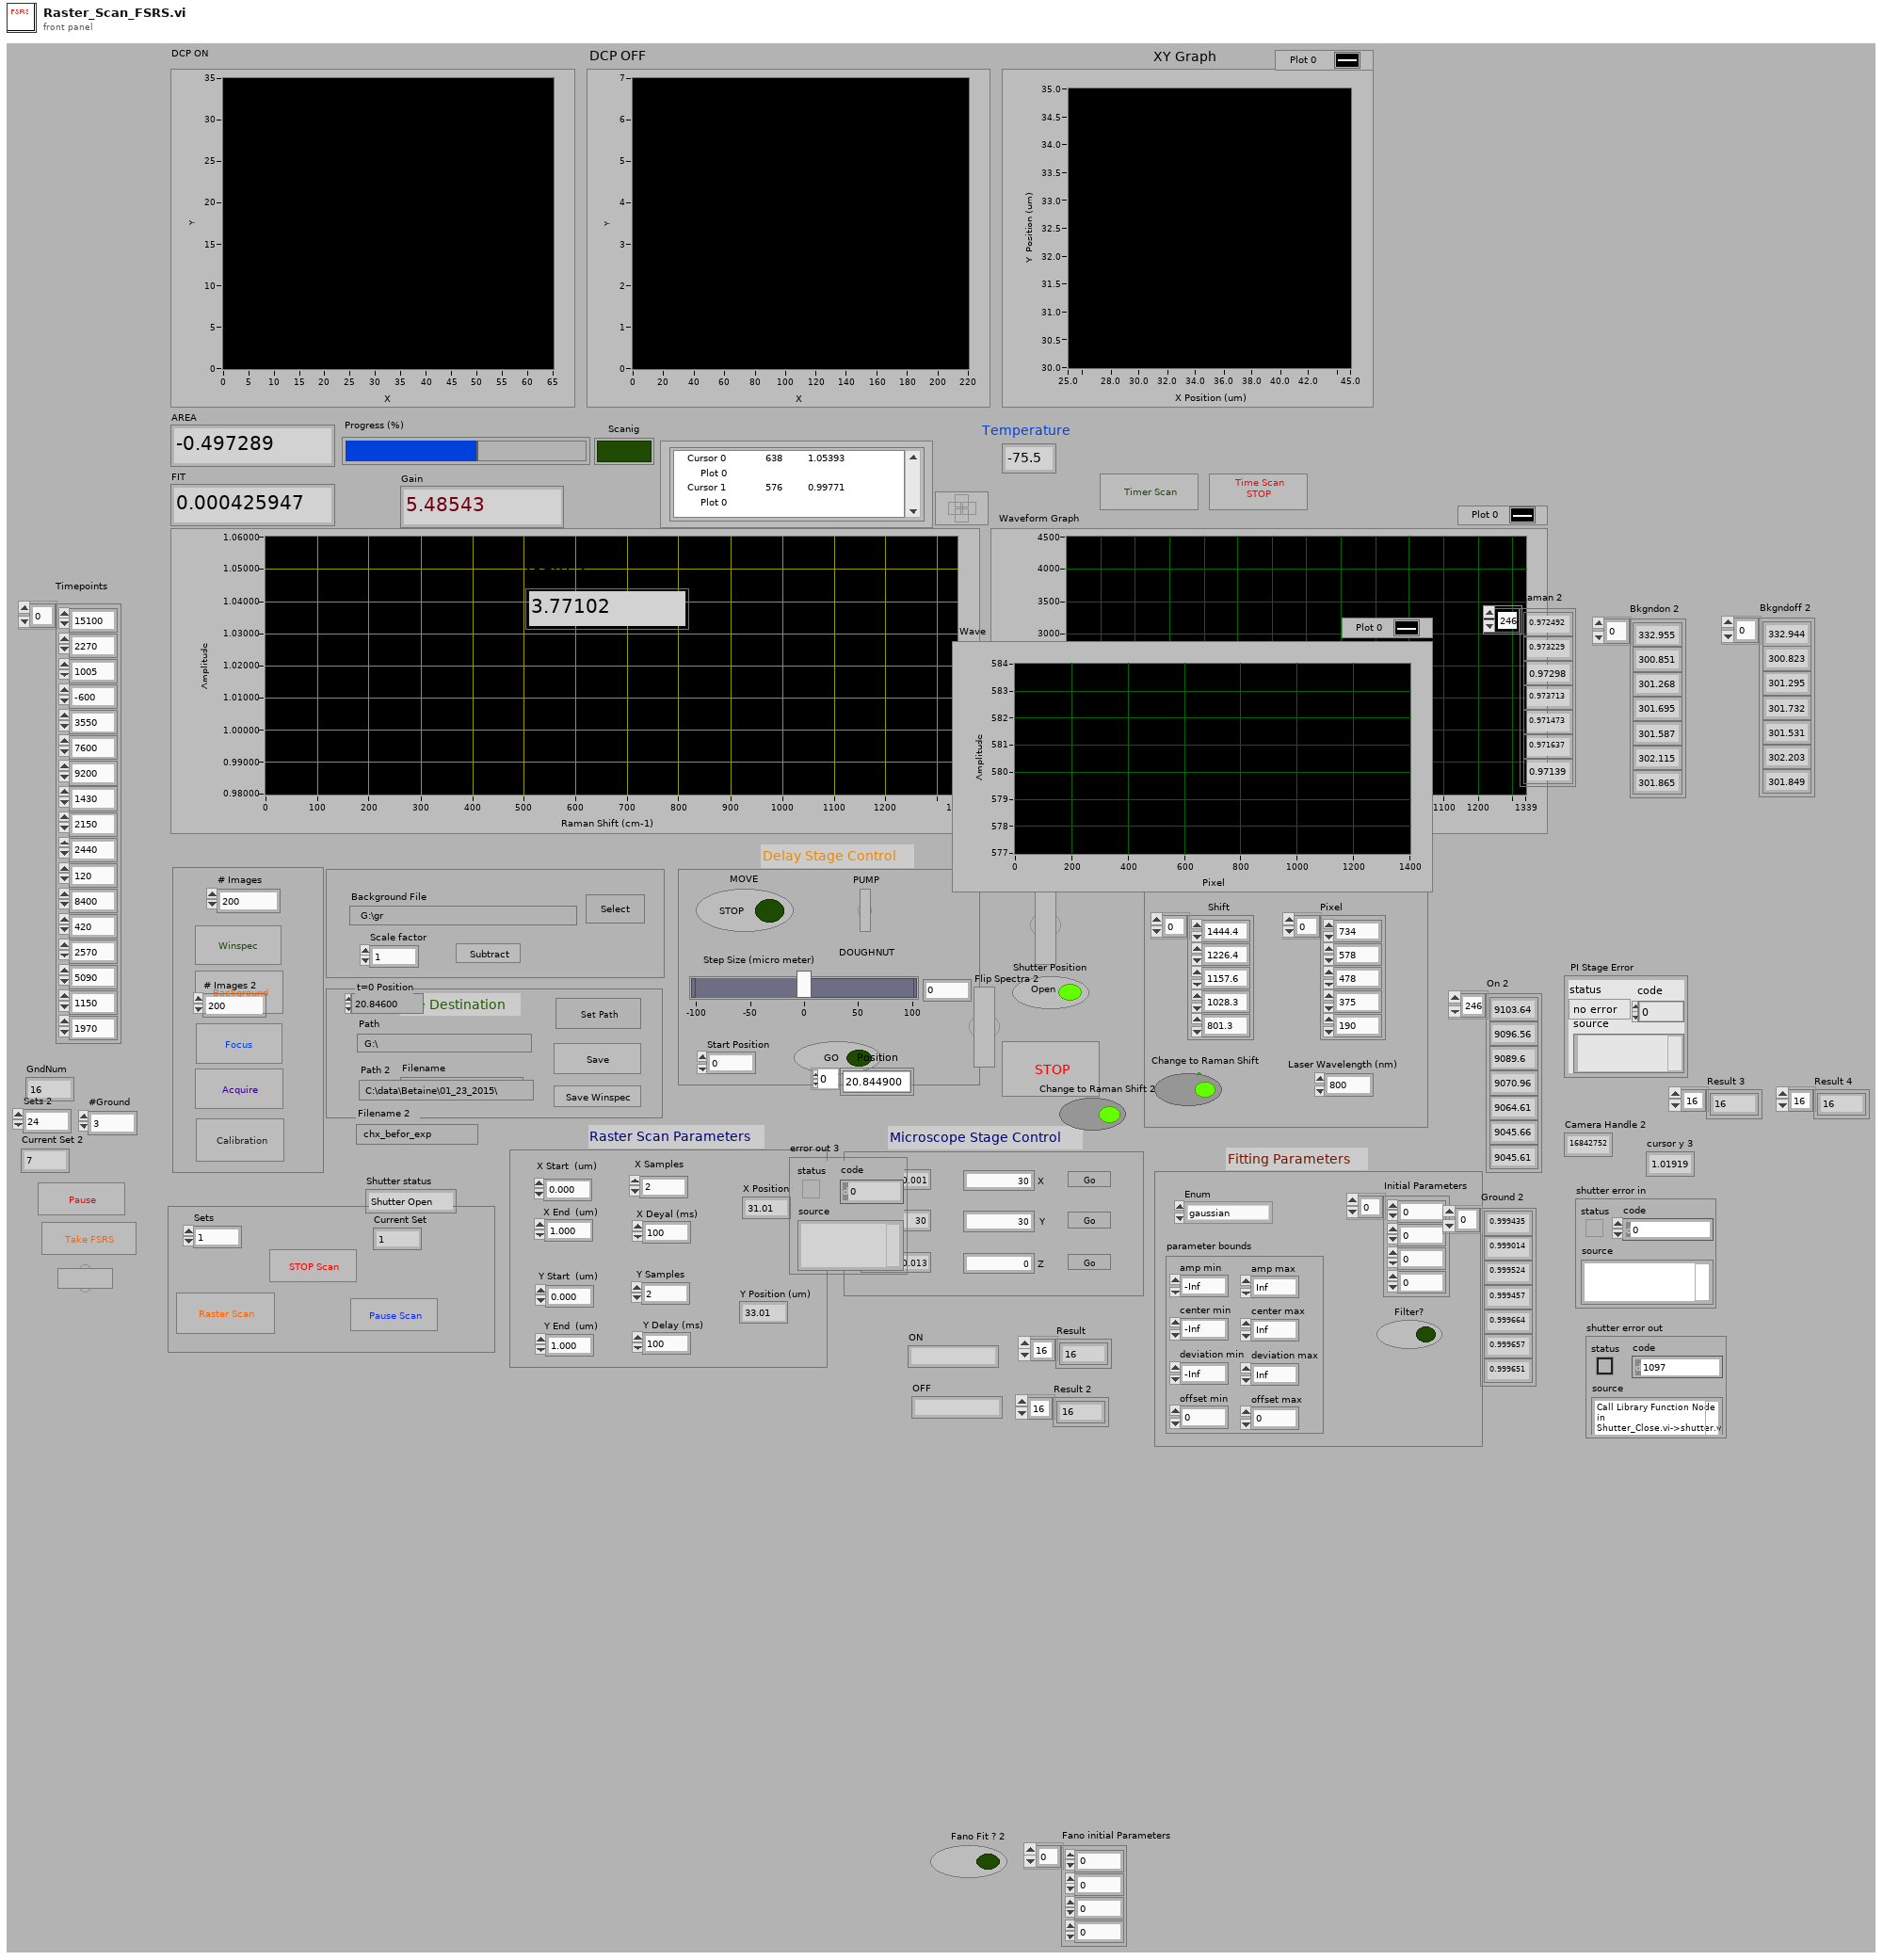
[diagram p1: front panel]
types:
  T1 = cluster{"amp min":dbl, "amp max":dbl, "center min":dbl, "center max":dbl, "deviation min":dbl, "deviation max":dbl, "offset min":dbl, "offset max":dbl}
  T2 = typedef "Control 2.ctl" = dbl[]
  T3 = enum8{"Enabled", "Disabled", "Disabled and Grayed Out"}
  T4 = cluster{"X start":u32, "X end":u32, "X Binning/Grouping":u32, "Y start":u32, "Y end":u32, "Y Binning/Grouping":u32}
  T5 = cluster{dbl[][], dbl[][], dbl[][], dbl[][], bool}
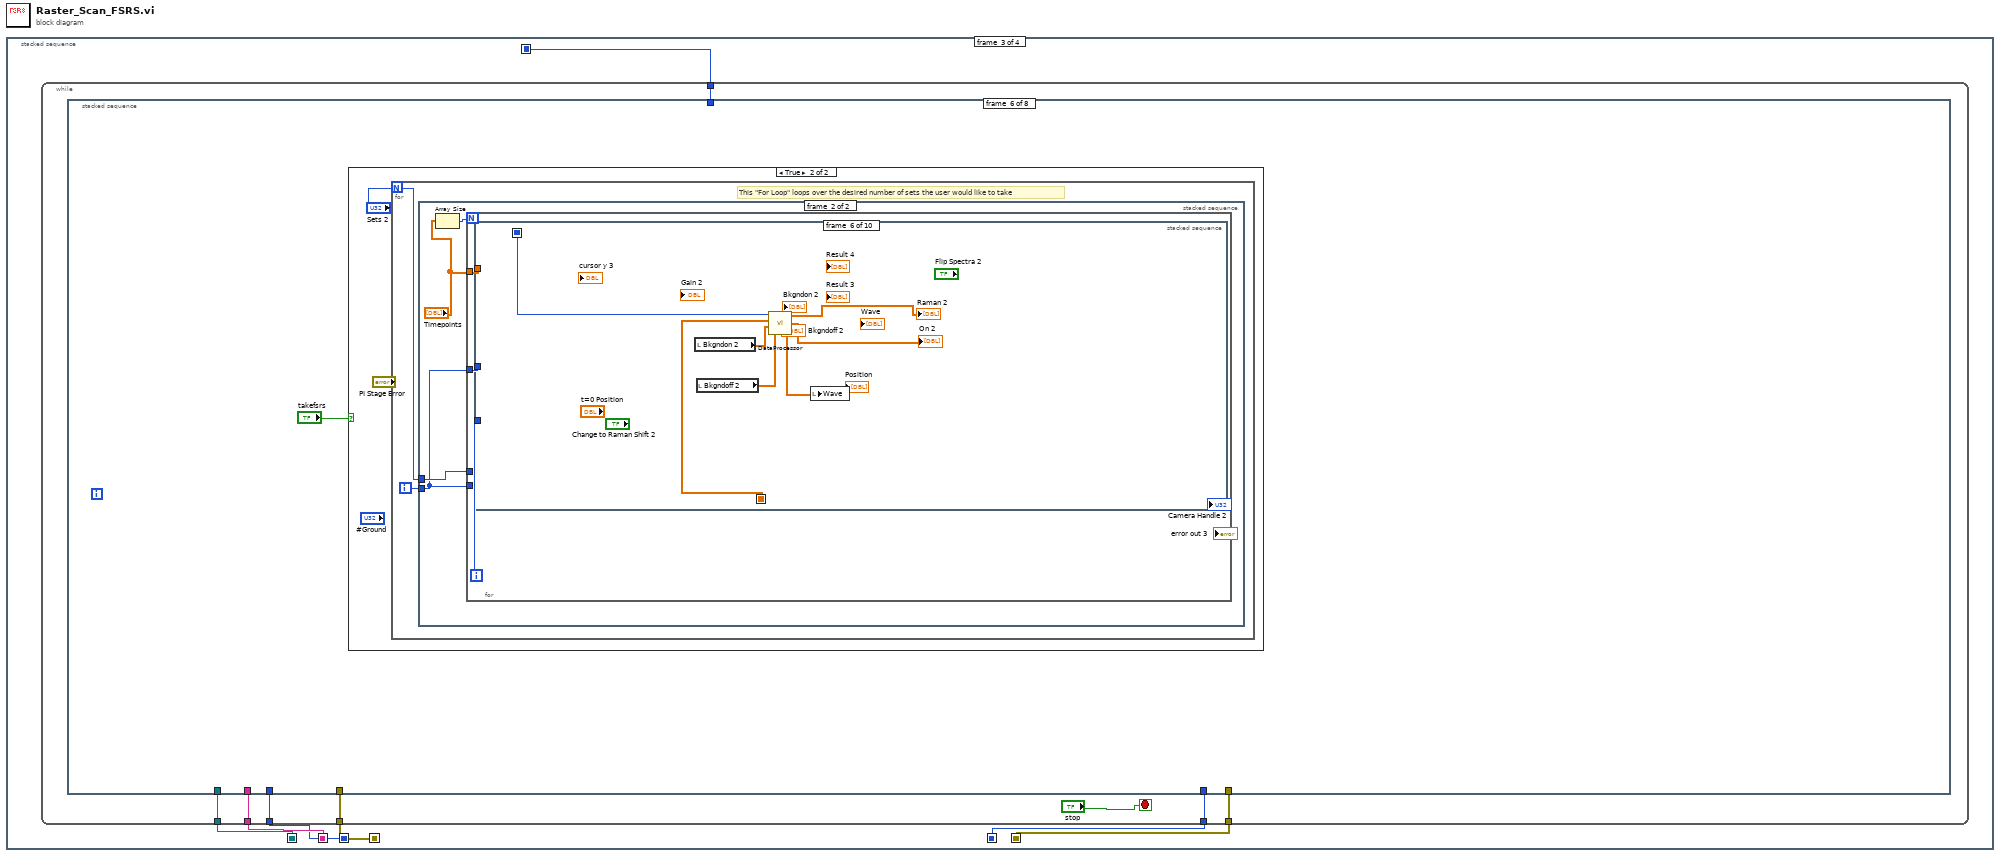
[diagram p0: block diagram]
diagram:
  n1 = stacked-sequence {
    seq-local: [w18 _ _ _] -> [_ _ w119 _]
    seq-local: [w17 _ _ _] -> [_ _ w118 _]
    seq-local: [w16 _ _ _] -> [_ _ w117 _]
    seq-local: [w15 _ _ _] -> [_ _ w116 _]
    seq-local: [w14 _ _ _] -> [_ _ w115 w1031]
    seq-local: [w13 _ _ _] -> [_ _ w114 _]
    seq-local: [w12 _ _ _] -> [_ _ w113 _]
    frame #0 {
      w10 = 1340
      w76 = 0
      w78 = 8
      # "4: shutter opened while waiting for trigger\n3: Shutter opened during entire acq sequence\n2:Shutter opened and closed for each exposure\n\nOther numbers: Time in ms to open and close"
      # "1 is for free run, 3 ext sync"
      # "Parameter id settings:\n119: enable custon timing for horizontal and vertical shift\n121:Parallel shift time override\n146: Skip serial register clean\n 4:  Set logic output to \"Not Ready\" (necessary for chopper sync)"
      # "Setting up the PIXIS and all the environment variables\nHave Renee fill in the rest."
      n2 = call "ExSubInitNOpenCam.vi"("error in (no error)"="error in") -> ("Camera Handle"=w91:u32, "error out"=w48:errorcluster)
      n3 = call <userlib>:"CameraGetDataDim.vi"("Camera Handle"=w91, "error in"=w48) -> ("Camera Handle"=w88:u32, "Xdim"=w90:u32, "Ydim"=w89:u32, "error out"=w87:errorcluster)
      n4 = global write "MaxX.vi" "X Max in"(w90) -> ()
      n5 = global write "MaxY.vi" "Max Y in"(w89) -> ()
      n6 = call "pico_init.vi"() -> ("error out 3"=w15:errorcluster, "ID"=w16:i32, "key"=w17:string, "CmdLib Out"=w18:refnum<k24>)  [unwired: 8 in]
      n7 = call <userlib>:"CameraSetTemp.vi"("error in (no error)"=w87, "Temperature"=-75, "Camera Handle"=w88) -> ("error out"=w84:errorcluster, "Camera Handle"=w85:u32)
      n8 = call <userlib>:"CameraADCset.vi"("ADC offset"=0, "Read Out port"=2, "error in (no error)"=w84, "ADC Gain"=1, "ADC Speed"=-2, "Camera Handle"=w85) -> ("error out"=w79:errorcluster, "Camera Handle"=w80:u32)
      n9 = Bundle(w78, w78, 100, w76, w76, w10) -> (w75:cluster{i32, i32, i32, i32, i32, i32})  [unwired: 1 in]
      n10 = call <userlib>:"CameraSetCustomChip.vi"("error in (no error)"=w79, "Custom Chip Settings"=w75, "Enable/Disable Custom Chip"=TRUE, "Camera Handle"=w80) -> ("error out"=w72:errorcluster, "Camera Handle"=w73:u32)
      n11 = call <userlib>:"CameraSkips.vi"("Camera Handle"=w73, "Minimum Block Size"=100, "Number of Minimum blocks"=1, "error in"=w72, "Type of Skips"=1) -> ("Camera Handle"=w67:u32, "error out"=w68:errorcluster)
      n12 = call "StandardInit.vi"() -> ("Outgoing Handle"=w14:i32)  [unwired: 1 in]
      n13 = call <userlib>:"CameraCleans.vi"("Camera Handle"=w67, "Number of Clears"=1, "Number of Strips Per Clear"=100, "error in"=w68, "Continuous Clears"=0) -> ("Camera Handle"=w62:u32, "error out"=w63:errorcluster)
      n14 = call <userlib>:"CameraTrigger.vi"("error in"=w63, "Trigger Edge"=1, "Timing Mode"=3, "Camera Handle"=w62) -> ("error out"=w40:errorcluster, "Camera Handle"=w39:u32)
      n15 = Bundle By Name(cluster=T4 {"X start"=0, "X end"=0, "X Binning/Grouping"=0, "Y start"=0, "Y end"=0, "Y Binning/Grouping"=0} ("ROI Params"), "X start"=u32 1, "X end"=u32 1340, "X Binning/Grouping"=u32 1, "Y start"=u32 1, "Y end"=u32 100, "Y Binning/Grouping"=u32 100) -> (w21:T4)
      n16 = call <userlib>:"CameraROI.vi"("error in"=w40, "ROI Params"=w21, "ROI Index"=1, "Camera Handle"=w39) -> ("error out"=w34:errorcluster, "Camera Handle"=w33:u32)
      n17 = call <userlib>:"CameraShutter.vi"("Camera Handle"=w33, "Shutter Comp Time: Pre Open"=0, "Shutter Comp Time: Post Open"=0, "error in"=w34, "Shutter State"=3) -> ("Camera Handle"=w32:u32, "error out"=w23:errorcluster)
      n18 = call <userlib>:"CameraSetVar.vi"("error in"=w23, "Value"=1.0, "Parameter ID"=119, "Camera Handle"=w32) -> ("error out"=w57:errorcluster, "CameraHandle"=w55:u32)
      n19 = call <userlib>:"CameraSetVar.vi"("error in"=w57, "Value"=3200.0, "Parameter ID"=121, "Camera Handle"=w55) -> ("error out"=w56:errorcluster, "CameraHandle"=w54:u32)
      n20 = call <userlib>:"CameraSetVar.vi"("error in"=w56, "Value"=1.0, "Parameter ID"=146, "Camera Handle"=w54) -> ("error out"=w28:errorcluster, "CameraHandle"=w27:u32)
      n21 = call <userlib>:"CameraSetVar.vi"("error in"=w28, "Value"=3.0, "Parameter ID"=4, "Camera Handle"=w27) -> ("error out"=w26:errorcluster, "CameraHandle"=w19:u32)
      n22 = call <userlib>:"ToolKitIsError.vi"("error in"=w26, "Reserved"=w19) -> ("error out"=w58:errorcluster, "Error Flag"=w59:bool)
      n23 = case shown="False" w59 {
        tunnel: w58 -> [_ w103]
        tunnel: [w102 w103] -> w20
        tunnel: w48 -> [w102 _]
        frame False {
        }
        frame True {
        }
      }
      n24 = while {
        tunnel: w20 -> [w100]
        tunnel: [w99] -> w36
        tunnel: w19 -> [w98]
        tunnel: [w97] -> w37
        stop <- w95 continue-if-true
        # "This loop makes sure the camera has cooled down completely"
        n25 = call <userlib>:"CameraGetTemp.vi"("Camera Handle"=w98, "error in (no error)"=w100) -> ("Camera Handle"=w97:u32, "Temperature"=w94:dbl, "error out"=w99:errorcluster)
        "Temperature" <- w94
        n26 = Wait Until Next ms Multiple(millisecond multiple=1000 ("ADC Gain")) -> ()  [unwired: 1 out]
        n27 = Greater?(x=w94, y=-75) -> (0:w95:bool)
      }
      "Camera Handle" <- w37
      "error out" <- w36
      n28 = for {
        N: w10 -> [_]
        tunnel: [w93] -> w11 mode=indexing
        i -> [w93]
      }
      n29 = local write "Result 2"(w11) -> ()
      n30 = local write "Result"(w11) -> ()
      n31 = call "Shutter_Init.vi"() -> ("error out"=w12:errorcluster, "ObjectPtr"=w13:i32)  [unwired: 2 in]
      n32 = property on="Callibration" class="Bool"("DisabledEnum"=T3."Disabled and Grayed Out" ("Disabled")) -> ()  [unwired: 2 in, 2 out]
      n33 = property on="Pause" class="Bool (strict)"("DisabledEnum"=T3."Disabled and Grayed Out" ("Disabled")) -> ()  [unwired: 2 in, 2 out]
      n34 = property on="winspec" class="Bool (strict)"("DisabledEnum"=T3."Disabled and Grayed Out" ("Disabled")) -> ()  [unwired: 2 in, 2 out]
      n35 = property on="Ruster Scan" class="Bool"("DisabledEnum"=T3."Disabled and Grayed Out" ("Disabled")) -> ()  [unwired: 2 in, 2 out]
      n36 = property on="Acquire" class="Bool"("DisabledEnum"=T3."Disabled and Grayed Out" ("Disabled")) -> ()  [unwired: 2 in, 2 out]
      n37 = property on="stop" class="Bool"("DisabledEnum"=T3."Disabled and Grayed Out" ("Disabled")) -> ()  [unwired: 2 in, 2 out]
      n38 = property on="STOP Scan" class="Bool"("DisabledEnum"=T3."Disabled and Grayed Out" ("Disabled")) -> ()  [unwired: 2 in, 2 out]
      n39 = property on="Focus" class="Bool (strict)"("DisabledEnum"=T3."Disabled and Grayed Out" ("Disabled")) -> ()  [unwired: 2 in, 2 out]
      n40 = property on="Bkgnd" class="Bool"("DisabledEnum"=T3."Disabled and Grayed Out" ("Disabled")) -> ()  [unwired: 2 in, 2 out]
    }
    frame #1 {
      n41 = property on="STOP Scan" class="Bool"("DisabledEnum"=T3."Enabled" ("Disabled")) -> ()  [unwired: 2 in, 2 out]
      n42 = property on="Pause" class="Bool (strict)"("DisabledEnum"=T3."Enabled" ("Disabled")) -> ()  [unwired: 2 in, 2 out]
      n43 = property on="stop" class="Bool"("DisabledEnum"=T3."Enabled" ("Disabled")) -> ()  [unwired: 2 in, 2 out]
      n44 = property on="Bkgnd" class="Bool"("DisabledEnum"=T3."Enabled" ("Disabled")) -> ()  [unwired: 2 in, 2 out]
      n45 = property on="Ruster Scan" class="Bool"("DisabledEnum"=T3."Enabled" ("Disabled")) -> ()  [unwired: 2 in, 2 out]
      n46 = property on="winspec" class="Bool (strict)"("DisabledEnum"=T3."Enabled" ("Disabled")) -> ()  [unwired: 2 in, 2 out]
      n47 = property on="Focus" class="Bool (strict)"("DisabledEnum"=T3."Enabled" ("Disabled")) -> ()  [unwired: 2 in, 2 out]
      n48 = property on="Acquire" class="Bool"("DisabledEnum"=T3."Enabled" ("Disabled")) -> ()  [unwired: 2 in, 2 out]
